vi "Quote and Escape JSON string.vi"(9 "Is System Encoding (T)":bool=TRUE, 11 "Plain Text":string) -> (3 "<JSON>":string caption="JSON string (quoted and escaped)")   [LabVIEW 2024, in "JSONtext.lvlib"]
uses:
  JSONtext.lvlib
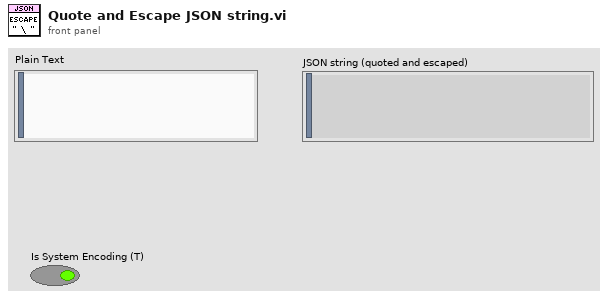
[diagram p1: front panel]
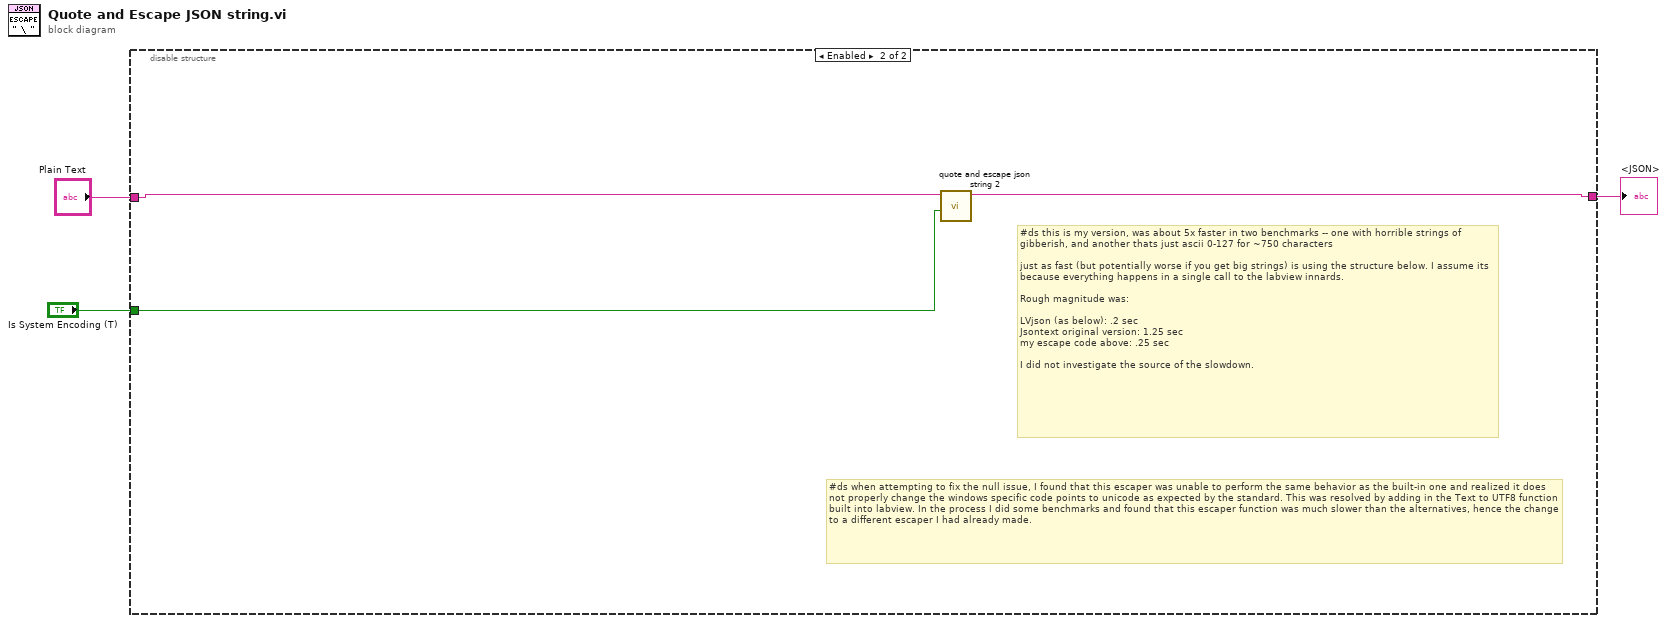
[diagram p0: block diagram]
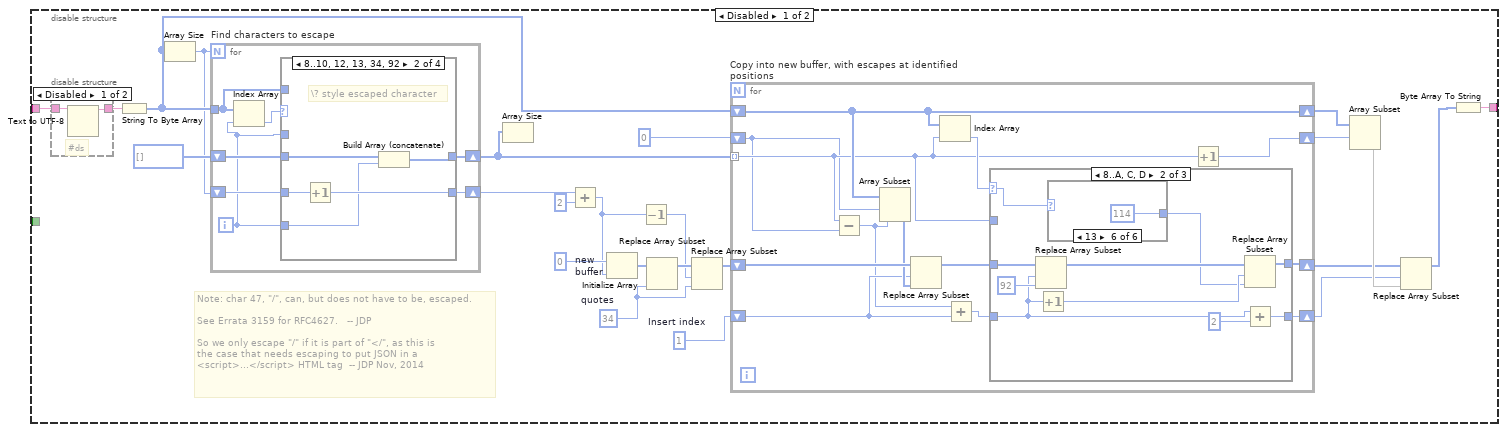
[diagram p2: hidden frame]
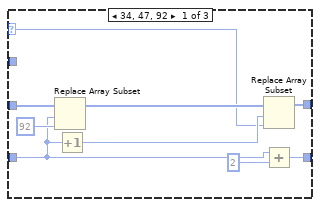
[diagram p4: hidden frame]
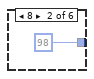
[diagram p6: hidden frame]
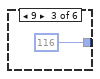
[diagram p7: hidden frame]
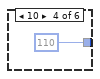
[diagram p8: hidden frame]
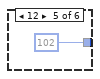
[diagram p9: hidden frame]
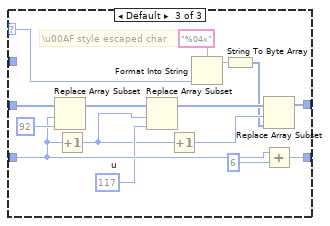
[diagram p10: hidden frame]
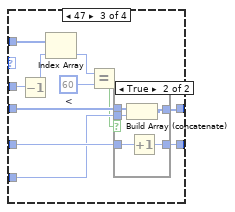
[diagram p12: hidden frame]
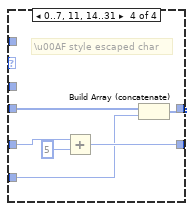
[diagram p14: hidden frame]
diagram:
  n1 = disable-structure shown="Enabled" {
    disable-tunnel: [w27 w122] -> w3
    disable-tunnel: "Plain Text" -> [w5 w123]
    disable-tunnel: "Is System Encoding (T)" -> [_ w121]
    frame Disabled {
      w8 = u8 34  # quotes
      w18 = 1  # Insert index
      # "Note: char 47, \"/\", can, but does not have to be, escaped.\n\nSee Errata 3159 for RFC4627.   -- JDP\n\nSo we only escape \"/\" if it is part of \"</\", as this is\nthe case that needs escaping to put JSON in a\n<script>...</script> HTML tag  -- JDP Nov, 2014"
      n2 = disable-structure shown="Disabled" {
        disable-tunnel: w5 -> [w29 w30]
        disable-tunnel: [w28 w30] -> w4
        frame Disabled {
          # "#ds"
          n3 = Text to UTF-8(11:w29) -> (3:w28:string)  [unwired: 2 in, 1 out]
        }
        frame Enabled {
        }
      }
      n4 = String To Byte Array(string=w4) -> (unsigned byte array=w22:u8[])
      n5 = Array Size(array=w22) -> (size(s)=w21:i32)
      n6 = for "Find characters to escape" {
        N: w21 -> [_]
        tunnel: w22 -> [w84]
        shift-right: [w88] -> w25
        shift-left: w21 -> [w89]
        shift-right: [w87] -> w23
        shift-left: i32[] [] -> [w86]
        i -> [w83]
        n7 = Index Array(array=w84, index=w83) -> (element=w85:u8)
        n8 = case shown="8..10, 12, 13, 34, 92" w85 {
          tunnel: w89 -> [w91 w96 w107 w117]
          tunnel: [w91 w95 w106 w120] -> w88
          tunnel: [w90 w94 w105 w119] -> w87
          tunnel: w86 -> [w90 w93 w104 w118]
          tunnel: w83 -> [_ w92 w103 w115]
          tunnel: w84 -> [_ _ w100 _]
          tunnel: w83 -> [_ _ w102 _]
          frame Default {
            # "Not escaped"
          }
          frame 8..10, 12, 13, 34, 92 {
            # "\\? style escaped character"
            n9 = Increment(x=w96) -> (x+1=w95:i32)
            n10 = Build Array (concatenate)(w93, w92) -> (w94:i32[])
          }
          frame 47 {
            w98 = u8 60  # <
            n11 = Decrement(x=w102) -> (x-1=w101:i32)
            n12 = Index Array(array=w100, index=w101) -> (element=w99:u8)
            n13 = Equal?(x=w99, y=w98) -> (x = y?=w97:bool)
            n14 = case shown="True" w97 {
              tunnel: w107 -> [w108 w114]
              tunnel: [w108 w113] -> w106
              tunnel: [w109 w112] -> w105
              tunnel: w104 -> [w109 w111]
              tunnel: w103 -> [_ w110]
              frame False {
              }
              frame True {
                n15 = Build Array (concatenate)(w111, w110) -> (w112:i32[])
                n16 = Increment(x=w114) -> (x+1=w113:i32)
              }
            }
          }
          frame 0..7, 11, 14..31 {
            # "\\u00AF style escaped char"
            n17 = Add(x=w117, y=5) -> (x+y=w120:i32)
            n18 = Build Array (concatenate)(w118, w115) -> (w119:i32[])
          }
        }
      }
      n19 = Array Size(array=w23) -> ()  [unwired: 1 out]
      n20 = Add(x=w25, y=2) -> (x+y=w10:i32)
      n21 = Initialize Array "new\nbuffer"(u8 0, w10) -> (w19:u8[])
      n22 = Decrement(x=w10) -> (x-1=w9:i32)
      n23 = Replace Array Subset(array=w19, new element=w8) -> (w12:u8[])  [unwired: 1 in]
      n24 = Replace Array Subset(array=w12, new element=w8, index=w9) -> (w11:u8[])
      n25 = for "Copy into new buffer, with escapes at identified positions" {
        tunnel: w23 -> [w33] mode=indexing
        shift-right: [w38] -> w15
        shift-left: w22 -> [w38]
        shift-right: [w37] -> w14
        shift-left: w18 -> [w36]
        shift-right: [w39] -> w16
        shift-left: w11 -> [w42]
        shift-right: [w31] -> w6
        shift-left: 0 -> [w32]
        n26 = Subtract(x=w33, y=w32) -> (x-y=w34:i32)
        n27 = Array Subset(array=w38, index=w32, length=w34) -> (w41:u8[])
        n28 = Replace Array Subset(array=w42, new element=w41, index=w36) -> (w40:u8[])
        n29 = Index Array(array=w38, index=w33) -> (element=w43:u8)
        n30 = Add(x=w34, y=w36) -> (x+y=w35:i32)
        n31 = case shown="8..A, C, D" w43 {
          selector: w43 -> [w48 w54 w74]
          tunnel: w40 -> [w52 w62 w82]
          tunnel: w33 -> [_ _ _]
          tunnel: [w47 w58 w80] -> w39
          tunnel: w35 -> [w44 w55 w77]
          tunnel: [w45 w56 w78] -> w37
          frame 34, 47, 92 {
            n32 = Replace Array Subset(array=w52, new element=u8 92 ("new element/subarray"), index=w44) -> (w50:u8[])
            n33 = Increment(x=w44) -> (x+1=w49:i32)
            n34 = Replace Array Subset(array=w50, new element=w48, index=w49) -> (w47:u8[])
            n35 = Add(x=w44, y=2) -> (x+y=w45:i32)
          }
          frame 8..10, 12, 13 {
            n36 = Replace Array Subset(array=w62, new element=u8 92 ("new element/subarray"), index=w55) -> (w60:u8[])
            n37 = Increment(x=w55) -> (x+1=w59:i32)
            n38 = case shown="13" w54 {
              tunnel: [_ u8 98 u8 116 u8 110 u8 102 u8 114] -> w53
              frame 0, Default {
              }
              frame 8 {
              }
              frame 9 {
              }
              frame 10 {
              }
              frame 12 {
              }
              frame 13 {
              }
            }
            n39 = Replace Array Subset(array=w60, new element=w53, index=w59) -> (w58:u8[])
            n40 = Add(x=w55, y=2) -> (x+y=w56:i32)
          }
          frame Default {
            w73 = u8 117  # u
            # "\\u00AF style escaped char"
            n41 = Replace Array Subset(array=w82, new element=u8 92 ("new element/subarray"), index=w77) -> (w72:u8[])
            n42 = Increment(x=w77) -> (x+1=w70:i32)
            n43 = Replace Array Subset(array=w72, new element=w73, index=w70) -> (w71:u8[])
            n44 = Increment(x=w70) -> (x+1=w69:i32)
            n45 = Format Into String(format string="%04x", w74) -> (resulting string=w75:string)  [unwired: 2 in, 1 out]
            n46 = String To Byte Array(string=w75) -> (unsigned byte array=w68:u8[])
            n47 = Replace Array Subset(array=w71, new element=w68, index=w69) -> (w80:u8[])
            n48 = Add(x=w77, y=6) -> (x+y=w78:i32)
          }
        }
        n49 = Increment(x=w33) -> (x+1=w31:i32)
      }
      n50 = Array Subset(array=w15, index=w6) -> (w17:u8[])  [unwired: 1 in]
      n51 = Replace Array Subset(array=w16, new element=w17, index=w14) -> (w24:u8[])
      n52 = Byte Array To String(unsigned byte array=w24) -> (string=w27:string)
    }
    frame Enabled {
      # "#ds when attempting to fix the null issue, I found that this escaper was unable to perform the same behavior as the built-in one and realized it does not properly change the windows specific code points to unicode as expected by the standard. This was resolved by adding in the Text to UTF8 function built into labview. In the process I did some benchmarks and found that this escaper function was much slower than the alternatives, hence the change to a different escaper I had already made."
      # "#ds this is my version, was about 5x faster in two benchmarks -- one with horrible strings of gibberish, and another thats just ascii 0-127 for ~750 characters\n\njust as fast (but potentially worse if you get big strings) is using the structure below. I assume its because everything happens in a single call to the labview innards.\n\nRough magnitude was:\n\nLVjson (as below): .2 sec\nJsontext original version: 1.25 sec\nmy escape code above: .25 sec\n\nI did not investigate the source of the slowdown."
      n53 = call "quote and escape json string 2.vi"("Is System Encoding (T)"=w121, "base string"=w123) -> ("String out"=w122:string)  [unwired: 9 in]
    }
  }
  "<JSON>" <- w3
